vi "queue_same_name.vi"() -> ()   [LabVIEW 2021]
panel:
  out "element 2":i32
  out "element":i32
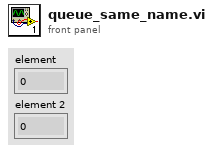
[diagram p1: front panel]
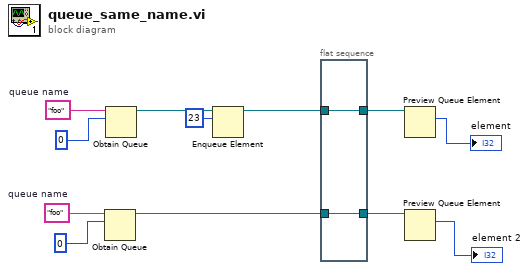
[diagram p0: block diagram]
diagram:
  w5 = "foo"  # queue name
  w12 = "foo"  # queue name
  n1 = Obtain Queue(name (unnamed)=w5, element data type=0) -> (queue out=w4:refnum<queue>)  [unwired: 3 in, 2 out]
  n2 = Obtain Queue(name (unnamed)=w12, element data type=0) -> (queue out=w10:refnum<queue>)  [unwired: 3 in, 2 out]
  n3 = Enqueue Element(queue=w10, element=23) -> (queue out=w9:refnum<queue>)  [unwired: 2 in, 2 out]
  n4 = flat-sequence {
    tunnel: w9 -> [w14]
    tunnel: [w14] -> w8
    tunnel: [w13] -> w3
    tunnel: w4 -> [w13]
    frame #0 {
    }
  }
  n5 = Preview Queue Element(queue=w8) -> (element=→"element":i32)  [unwired: 2 in, 3 out]
  n6 = Preview Queue Element(queue=w3) -> (element=→"element 2":i32)  [unwired: 2 in, 3 out]
